vi "rqcAlice Delay Line Test (Low Level Example).vi"() -> ()   [LabVIEW 2018]
uses:
  FPGA/Alice/Custom Controls/Phase Modulator/rqcAlice Mod.Config.ctl
  Custom Controls/rqcAlice States.ctl
  FPGA/Alice/Custom Controls/Main State Machine/rqcAlice DAC Clock Positions.ctl
  Shared/Shared FPGA Lib/Shared Logic/Custom Controls/rqc Random Generator.parameters.ctl
  Shared/Shared FPGA Lib/Shared Logic/Custom Controls/rqc Random Generator.value type.ctl
  Shared/Shared Host Lib/rqc ServiceNET/Custom Controls/rqc ServiceNET command.ctl
  Shared/Shared Host Lib/rqc ServiceNET/Alice/Custom Controls/rqcAlice ServiceNET control.ctl
  <vilib>/FPGAPlugInAG/PCI-7811R/niLvFpga_Open_PCI-7811R.vi
  <vilib>/rvi/interface/common/dynamic/niFpgaDynamicAddResources.vi
  <vilib>/FPGAPlugInAG/Dynamic/niLvFpga_Close_Dynamic.vi
  <vilib>/rvi/interface/nirviOpenFPGA/nirviOpenFPGA.xnode
  FPGA Bitfiles/rqcAlice FPGA (7811R) v 2.3.0.lvbitx
  <vilib>/rvi/interface/nirviCloseFPGA/nirviCloseFPGA.xnode
panel:
  in  "Attenuation, dB":fxp<+,7,6>
  in  "SD/Coax Select":bool
  in  "RndGen.parameters":T1={"value type"=enum."constant", "constant"=150, "num of levels"=0, "levels values"=[0, 0, 0, 0]}
  in  "DAC Clock params":T3=[18, 38]
  out "XY Graph":T4(graph)={"appended array"=[49350.0, 49351.0, 49352.0, 49353.0, 49354.0, 49355.0, 49356.0, 49357.0, 49358.0, 49359.0, 49360.0, 49361.0, 49362.0, 49363.0, 49364.0, 49365.0, 49366.0, 49367.0, 49368.0, 49369.0, 49370.0, 49371.0, 49372.0, 49373.0, 49374.0, 49375.0, 49376.0, 49377.0, 49378.0, 49379.0, 49380.0, 49381.0, 49382.0, 49383.0, 49384.0, 49385.0, 49386.0, 49387.0, 49388.0, 49389.0, 49390.0, 49391.0, 49392.0, 49393.0, 49394.0, 49395.0, 49396.0, 49397.0, 49398.0, 49399.0, 49400.0, 49401.0, 49402.0, 49403.0, 49404.0, 49405.0, 49406.0, 49407.0, 49408.0, 49409.0, 49410.0, 49411.0, 49412.0, 49413.0, 49414.0, 49415.0, 49416.0, 49417.0, 49418.0, 49419.0, 49420.0, 49421.0, 49422.0, 49423.0, 49424.0, 49425.0, 49426.0, 49427.0, 49428.0, 49429.0, 49430.0, 49431.0, 49432.0, 49433.0, 49434.0, 49435.0], "appended array"=[4.0, 12.0, 24.0, 27.0, 45.0, 53.0, 39.0, 47.0, 36.0, 40.0, 40.0, 34.0, 37.0, 25.0, 9.0, 7.0, 2.0, 0.0, 0.0, 5.0, 8.0, 17.0, 20.0, 30.0, 49.0, 49.0, 43.0, 39.0, 48.0, 46.0, 47.0, 34.0, 29.0, 19.0, 9.0, 9.0, 1.0, 4.0, 3.0, 7.0, 5.0, 9.0, 23.0, 38.0, 37.0, 54.0, 30.0, 46.0, 51.0, 40.0, 47.0, 37.0, 33.0, 8.0, 5.0, 4.0, 3.0, 1.0, 3.0, 0.0, 3.0, 8.0, 15.0, 26.0, 33.0, 39.0, 45.0, 48.0, 54.0, 48.0, 44.0, 41.0, 43.0, 33.0, 20.0, 12.0, 9.0, 3.0, 2.0, 3.0, 5.0, 11.0, 19.0, 25.0, 34.0]}
  out "Delay Line Value":u32=49435
  in  "Delay Line Delta":u32=1
  in  "Delay Line max":u32=49450
  in  "Delay Line min":u32=49350
  out "error out":errorcluster
  in  "Stop":bool
  out "connected?":bool
  in  "port":u16=5020
  out "Current State":T5=enum."App.Stop"
  in  "Modulator config":T6={"mod.on"=9, "mod.off"=2}
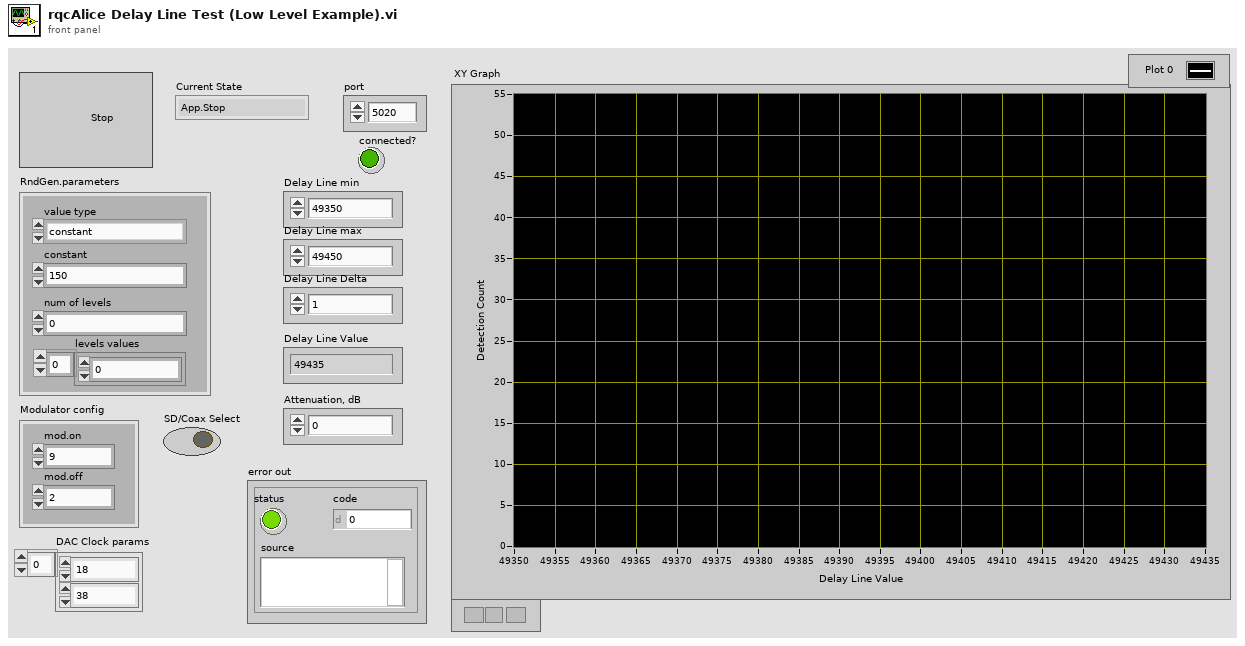
[diagram p1: front panel]
types:
  T1 = typedef "rqc Random Generator.parameters.ctl" = cluster{"value type":T2, "constant":u16, "num of levels":u16, "levels values":u16[]}
  T2 = typedef "rqc Random Generator.value type.ctl" = enum16{"random value", "constant"}
  T3 = typedef "rqcAlice DAC Clock Positions.ctl" = u8[]
  T4 = cluster{"appended array":dbl[], "appended array":dbl[]}
  T5 = typedef "rqcAlice States.ctl" = enum16{"HW.configure", "HW.meas", "NET.create", "NET.connect", "NET.readCommand", "NET.sendCommand", "NET.readData", "NET.close", "Meas.Start", "Meas.NextStep", "Meas.restart", "Meas.Done", "App.HandleEvent", "App.HandleError", "App.Stop"}
  T6 = typedef "rqcAlice Mod.Config.ctl" = cluster{"mod.on":u8, "mod.off":u8}
  T7 = typedef "rqc ServiceNET command.ctl" = enum8{"NONE", "READY", "START", "PING"}
  T8 = typedef "rqcAlice ServiceNET control.ctl" = cluster{"connection ID":refnum<k5>, "port":u16, "connected?":bool}
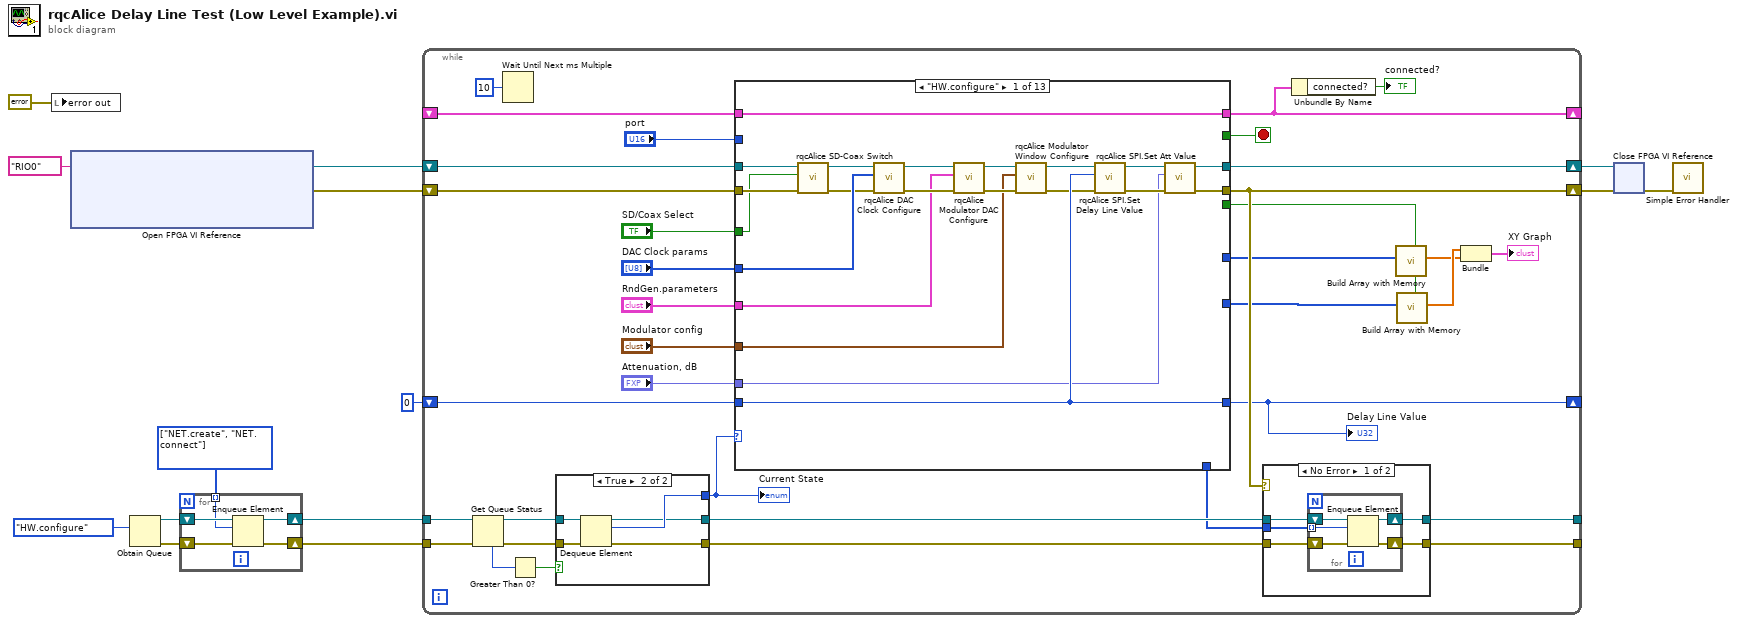
[diagram p0: block diagram]
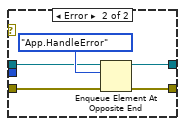
[diagram p2: hidden frame]
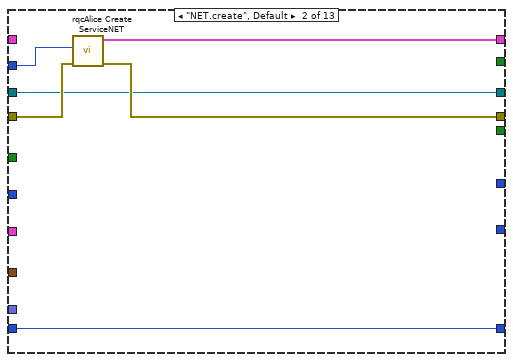
[diagram p3: hidden frame]
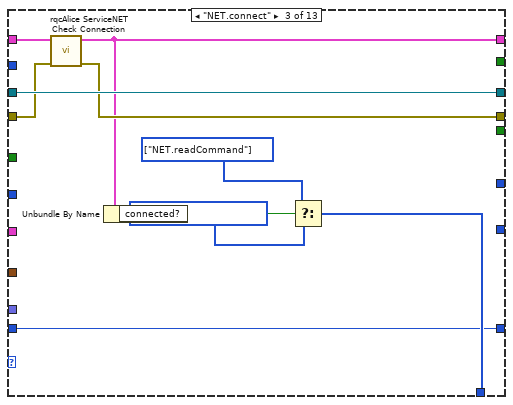
[diagram p4: hidden frame]
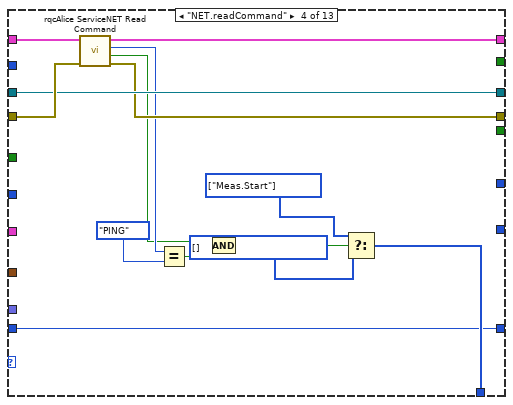
[diagram p5: hidden frame]
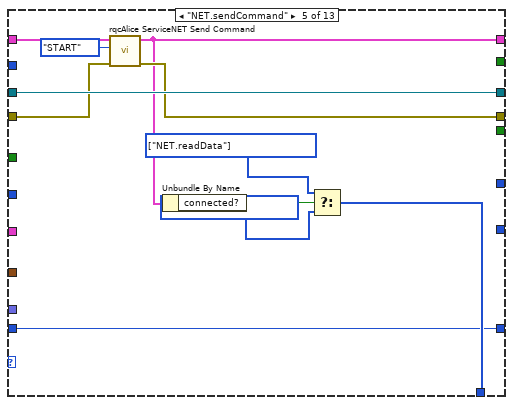
[diagram p6: hidden frame]
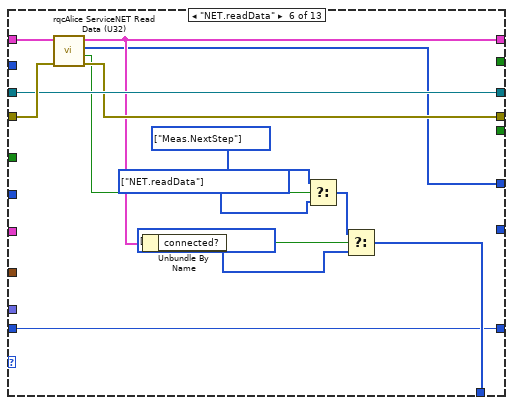
[diagram p7: hidden frame]
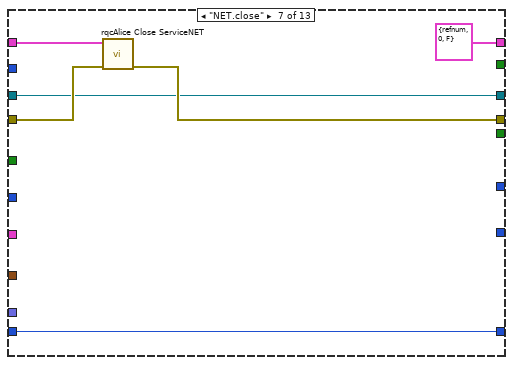
[diagram p8: hidden frame]
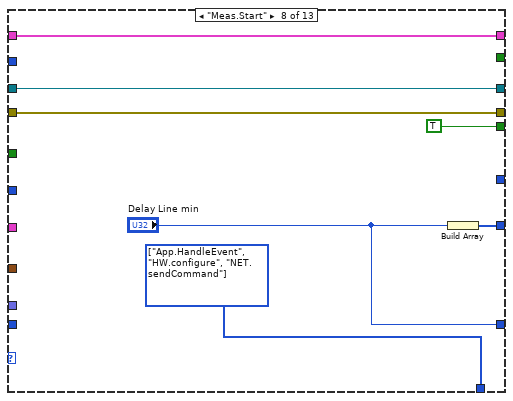
[diagram p9: hidden frame]
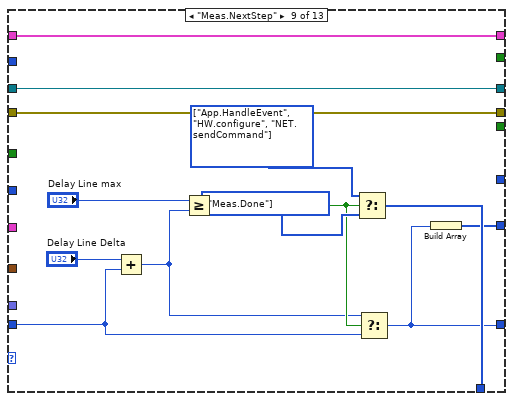
[diagram p10: hidden frame]
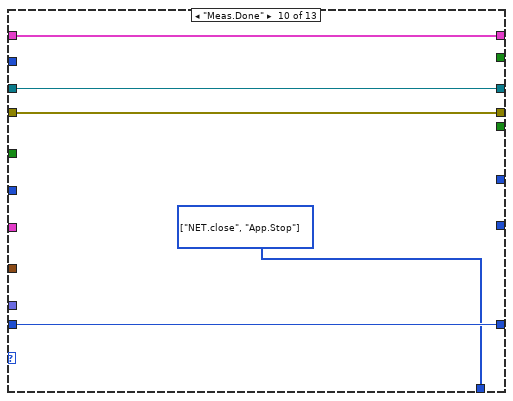
[diagram p11: hidden frame]
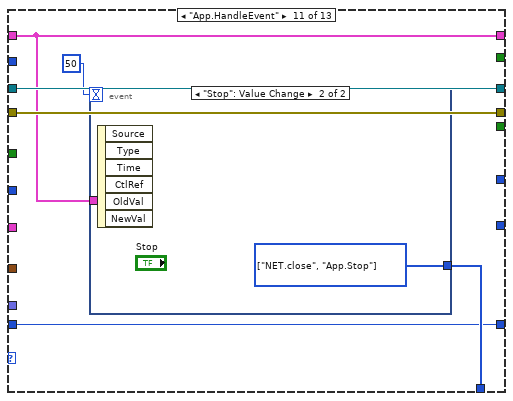
[diagram p12: hidden frame]
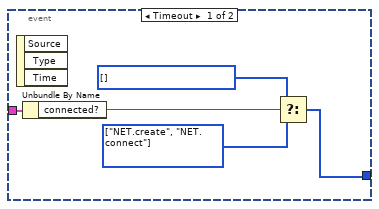
[diagram p13: hidden frame]
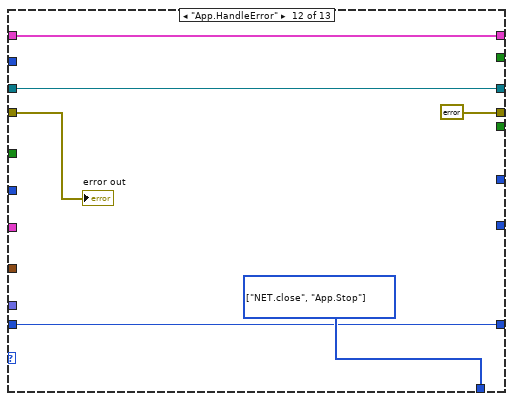
[diagram p14: hidden frame]
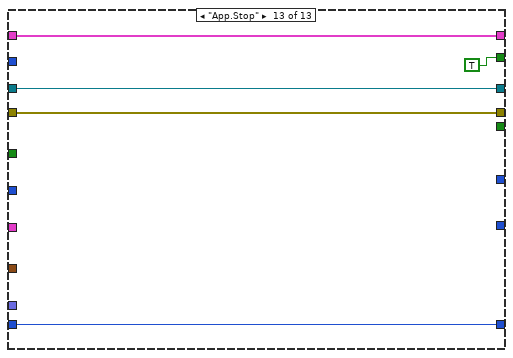
[diagram p15: hidden frame]
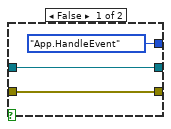
[diagram p16: hidden frame]
diagram:
  w6 = T5[] [enum."NET.create", enum."NET.connect"] items=["HW.configure", "HW.meas", "NET.create", "NET.connect", "NET.readCommand", "NET.sendCommand", "NET.readData", "NET.close", "Meas.Start", "Meas.NextStep", "Meas.restart", "Meas.Done", "App.HandleEvent", "App.HandleError", "App.Stop"]
  n1 = local write "error out"(errorcluster {"status"=FALSE, "code"=0, "source"=""} ("error out")) -> ()
  n2 = xnode "Open FPGA VI Reference"("resource name"=tag "RIO0") -> ("FPGA VI Reference Out"=w13:refnum<k20>, "error out"=w12:errorcluster)  [unwired: 1 in]
  n3 = Obtain Queue(element data type=rqcAlice_States."HW.configure" ("rqcAlice States")) -> (queue out=w8:refnum<queue>, error out=w7:errorcluster)  [unwired: 4 in, 1 out]
  n4 = for {
    shift-right: [w17] -> w5
    shift-left: w8 -> [w19]
    shift-right: [w16] -> w4
    shift-left: w7 -> [w18]
    tunnel: w6 -> [w15] mode=indexing
    n5 = Enqueue Element(queue=w19, element=w15, error in (no error)=w18) -> (queue out=w17:refnum<queue>, error out=w16:errorcluster)  [unwired: 1 in, 1 out]
  }
  n6 = while {
    tunnel: w5 -> [w50]
    shift-right: [w51] -> w11
    shift-left: w13 -> [w54]
    shift-right: [w43] -> w10
    shift-left: w12 -> [w53]
    tunnel: w4 -> [w49]
    tunnel: [w40] -> _
    tunnel: [w39] -> _
    shift-right: [w35] -> _
    shift-left: _ -> [w37]
    shift-right: [w29] -> _
    shift-left: u32 0 ("Delay Line min") -> [w31]
    stop <- w33 stop-if-true
    n7 = Get Queue Status(queue=w50, error in (no error)=w49) -> (queue out=w46:refnum<queue>, error out=w45:errorcluster, # elements in queue=w48:i32)  [unwired: 1 in, 5 out]
    n8 = Wait Until Next ms Multiple(millisecond multiple=u32 10) -> ()  [unwired: 1 out]
    n9 = Greater Than 0?(x=w48) -> (x > 0?=w47:bool)
    n10 = case shown="True" w47 {
      tunnel: w46 -> [w201 w207]
      tunnel: w45 -> [w200 w206]
      tunnel: [rqcAlice_States."App.HandleEvent" ("rqcAlice States") w205] -> w44
      tunnel: [w201 w204] -> w42
      tunnel: [w200 w203] -> w41
      frame False {
      }
      frame True {
        n11 = Dequeue Element(queue=w207, error in (no error)=w206) -> (queue out=w204:refnum<queue>, element=w205:T5, error out=w203:errorcluster)  [unwired: 1 in, 1 out]
      }
    }
    "Current State" <- w44
    n12 = case shown="\"HW.configure\"" w44 {
      tunnel: w54 -> [w82 w93 w106 w117 w131 w143 w147 w157 w170 w175 w182 w193 w198]
      tunnel: w53 -> [w81 w95 w104 w119 w129 w144 w150 w156 w169 w174 w181 w192 w197]
      tunnel: "Modulator config" -> [w86 _ _ _ _ _ _ _ _ _ _ _ _]
      tunnel: [w73 w93 w106 w117 w131 w143 w147 w157 w170 w175 w182 w193 w198] -> w51
      tunnel: [w71 w94 w103 w116 w128 w142 w149 w156 w169 w174 w181 errorcluster {"status"=FALSE, "code"=0, "source"=""} ("error out") w197] -> w43
      tunnel: [_ _ w99 w108 w122 w134 _ w155 w165 w172 w178 w190 _] -> w38
      tunnel: [w85 w96 w102 w118 w126 w141 T8 {"connection ID"=refnum, "port"=0, "connected?"=FALSE} ("rqcAlice ServiceNET out") w158 w171 w176 w179 w194 w196] -> w35
      tunnel: w37 -> [w85 _ w105 w120 w130 w145 w151 w158 w171 w176 w179 w194 w196]
      tunnel: "port" -> [_ w92 _ _ _ _ _ _ _ _ _ _ _]
      tunnel: [_ _ _ _ _ _ _ _ _ _ _ _ TRUE] -> w33
      tunnel: w31 -> [w76 w91 w97 w107 w121 w133 w146 _ w161 w173 w177 w189 w195]
      tunnel: [w76 w91 w97 w107 w121 w133 w146 "Delay Line min" w160 w173 w177 w189 w195] -> w29
      tunnel: [_ _ _ _ _ w132 _ _ _ _ _ _ _] -> w30
      tunnel: [_ _ _ _ _ _ _ w152 w159 _ _ _ _] -> w28
      tunnel: [_ _ _ _ _ _ _ TRUE _ _ _ _ _] -> w27
      tunnel: "DAC Clock params" -> [w84 _ _ _ _ _ _ _ _ _ _ _ _]
      tunnel: "RndGen.parameters" -> [w83 _ _ _ _ _ _ _ _ _ _ _ _]
      tunnel: "SD/Coax Select" -> [w78 _ _ _ _ _ _ _ _ _ _ _ _]
      tunnel: "Attenuation, dB" -> [w70 _ _ _ _ _ _ _ _ _ _ _ _]
      frame "HW.configure" {
        n13 = call "rqcAlice SD-Coax Switch.vi"("error in"=w81, "SD/Coax Select"=w78, "Alice FPGA Reference In"=w82) -> ("error out"=w79:errorcluster, "Alice FPGA Reference Out"=w80:refnum<k20>)  [unwired: 7 in]
        n14 = call "rqcAlice DAC Clock Configure.vi"("error in"=w79, "DAC Clock params"=w84, "Alice FPGA Reference In"=w80) -> ("error out"=w89:errorcluster, "Alice FPGA Reference Out"=w90:refnum<k20>)  [unwired: 7 in]
        n15 = call "rqcAlice Modulator DAC Configure.vi"("error in"=w89, "RndGen.parameters"=w83, "Alice FPGA Reference In"=w90) -> ("error out"=w87:errorcluster, "Alice FPGA Reference Out"=w88:refnum<k20>)  [unwired: 7 in]
        n16 = call "rqcAlice Modulator Window Configure.vi"("error in"=w87, "Modulator config"=w86, "Alice FPGA Reference In"=w88) -> ("error out"=w75:errorcluster, "Alice FPGA Reference Out"=w77:refnum<k20>)  [unwired: 7 in]
        n17 = call "rqcAlice SPI.Set Delay Line Value.vi"("error in"=w75, "Delay Line Value"=w76, "Alice FPGA Reference In"=w77) -> ("error out"=w72:errorcluster, "Alice FPGA Reference Out"=w74:refnum<k20>)  [unwired: 7 in]
        n18 = call "rqcAlice SPI.Set Att Value.vi"("error in"=w72, "Attenuation, dB"=w70, "Alice FPGA Reference In"=w74) -> ("error out"=w71:errorcluster, "Alice FPGA Reference Out"=w73:refnum<k20>)  [unwired: 7 in]
      }
      frame "NET.create", Default {
        n19 = call "rqcAlice Create ServiceNET.vi"("error in"=w95, "port"=w92) -> ("error out"=w94:errorcluster, "rqcAlice ServiceNET control"=w96:T8)  [unwired: 8 in]
      }
      frame "NET.connect" {
        w98 = T5[] [] items=["HW.configure", "HW.meas", "NET.create", "NET.connect", "NET.readCommand", "NET.sendCommand", "NET.readData", "NET.close", "Meas.Start", "Meas.NextStep", "Meas.restart", "Meas.Done", "App.HandleEvent", "App.HandleError", "App.Stop"] ("f")
        w100 = T5[] [enum."NET.readCommand"] items=["HW.configure", "HW.meas", "NET.create", "NET.connect", "NET.readCommand", "NET.sendCommand", "NET.readData", "NET.close", "Meas.Start", "Meas.NextStep", "Meas.restart", "Meas.Done", "App.HandleEvent", "App.HandleError", "App.Stop"]
        n20 = call "rqcAlice ServiceNET Check Connection.vi"("error in"=w104, "rqcAlice ServiceNET in"=w105) -> ("error out"=w103:errorcluster, "rqcAlice ServiceNET out"=w102:T8)  [unwired: 8 in]
        n21 = Unbundle By Name(w102) -> ("connected?"=w101:bool)
        n22 = Select(t=w100, s=w101, f=w98) -> (s? t:f=w99:T5[])
      }
      frame "NET.readCommand" {
        w109 = T5[] [] items=["HW.configure", "HW.meas", "NET.create", "NET.connect", "NET.readCommand", "NET.sendCommand", "NET.readData", "NET.close", "Meas.Start", "Meas.NextStep", "Meas.restart", "Meas.Done", "App.HandleEvent", "App.HandleError", "App.Stop"] ("f")
        w110 = T5[] [enum."Meas.Start"] items=["HW.configure", "HW.meas", "NET.create", "NET.connect", "NET.readCommand", "NET.sendCommand", "NET.readData", "NET.close", "Meas.Start", "Meas.NextStep", "Meas.restart", "Meas.Done", "App.HandleEvent", "App.HandleError", "App.Stop"] ("f")
        n23 = call "rqcAlice ServiceNET Read Command.vi"("error in"=w119, "rqcAlice ServiceNET in"=w120) -> ("error out"=w116:errorcluster, "cmd valid"=w112:bool, "command"=w114:T7, "rqcAlice ServiceNET out"=w118:T8)  [unwired: 6 in]
        n24 = Equal?(x=w114, y=rqc_ServiceNET_command."PING" ("command")) -> (x = y?=w113:bool)
        n25 = Compound Arithmetic op=AND(w112, w113) -> (w111:bool)
        n26 = Select(t=w110, s=w111, f=w109) -> (s? t:f=w108:T5[])
      }
      frame "NET.sendCommand" {
        w123 = T5[] [] items=["HW.configure", "HW.meas", "NET.create", "NET.connect", "NET.readCommand", "NET.sendCommand", "NET.readData", "NET.close", "Meas.Start", "Meas.NextStep", "Meas.restart", "Meas.Done", "App.HandleEvent", "App.HandleError", "App.Stop"] ("f")
        w124 = T5[] [enum."NET.readData"] items=["HW.configure", "HW.meas", "NET.create", "NET.connect", "NET.readCommand", "NET.sendCommand", "NET.readData", "NET.close", "Meas.Start", "Meas.NextStep", "Meas.restart", "Meas.Done", "App.HandleEvent", "App.HandleError", "App.Stop"] ("f")
        n27 = call "rqcAlice ServiceNET Send Command.vi"("error in"=w129, "command"=rqc_ServiceNET_command."START", "rqcAlice ServiceNET in"=w130) -> ("error out"=w128:errorcluster, "rqcAlice ServiceNET out"=w126:T8)  [unwired: 7 in]
        n28 = Unbundle By Name(w126) -> ("connected?"=w125:bool)
        n29 = Select(t=w124, s=w125, f=w123) -> (s? t:f=w122:T5[])
      }
      frame "NET.readData" {
        w135 = T5[] [] items=["HW.configure", "HW.meas", "NET.create", "NET.connect", "NET.readCommand", "NET.sendCommand", "NET.readData", "NET.close", "Meas.Start", "Meas.NextStep", "Meas.restart", "Meas.Done", "App.HandleEvent", "App.HandleError", "App.Stop"] ("f")
        w140 = T5[] [enum."Meas.NextStep"] items=["HW.configure", "HW.meas", "NET.create", "NET.connect", "NET.readCommand", "NET.sendCommand", "NET.readData", "NET.close", "Meas.Start", "Meas.NextStep", "Meas.restart", "Meas.Done", "App.HandleEvent", "App.HandleError", "App.Stop"] ("t")
        w138 = T5[] [enum."NET.readData"] items=["HW.configure", "HW.meas", "NET.create", "NET.connect", "NET.readCommand", "NET.sendCommand", "NET.readData", "NET.close", "Meas.Start", "Meas.NextStep", "Meas.restart", "Meas.Done", "App.HandleEvent", "App.HandleError", "App.Stop"] ("f")
        n30 = call "rqcAlice ServiceNET Read Data (U32).vi"("error in"=w144, "rqcAlice ServiceNET in"=w145) -> ("error out"=w142:errorcluster, "data valid"=w139:bool, "data"=w132:u32[], "rqcAlice ServiceNET out"=w141:T8)  [unwired: 6 in]
        n31 = Unbundle By Name(w141) -> ("connected?"=w137:bool)
        n32 = Select(t=w140, s=w139, f=w138) -> (s? t:f=w136:T5[])
        n33 = Select(t=w136, s=w137, f=w135) -> (s? t:f=w134:T5[])
      }
      frame "NET.close" {
        n34 = call "rqcAlice Close ServiceNET.vi"("error in"=w150, "rqcAlice ServiceNET in"=w151) -> ("error out"=w149:errorcluster)  [unwired: 9 in]
      }
      frame "Meas.Start" {
        w155 = T5[] [enum."App.HandleEvent", enum."HW.configure", enum."NET.sendCommand"] items=["HW.configure", "HW.meas", "NET.create", "NET.connect", "NET.readCommand", "NET.sendCommand", "NET.readData", "NET.close", "Meas.Start", "Meas.NextStep", "Meas.restart", "Meas.Done", "App.HandleEvent", "App.HandleError", "App.Stop"] ("f")
        n35 = Build Array("Delay Line min") -> (w152:u32[])
      }
      frame "Meas.NextStep" {
        w164 = T5[] [enum."Meas.Done"] items=["HW.configure", "HW.meas", "NET.create", "NET.connect", "NET.readCommand", "NET.sendCommand", "NET.readData", "NET.close", "Meas.Start", "Meas.NextStep", "Meas.restart", "Meas.Done", "App.HandleEvent", "App.HandleError", "App.Stop"] ("f")
        w166 = T5[] [enum."App.HandleEvent", enum."HW.configure", enum."NET.sendCommand"] items=["HW.configure", "HW.meas", "NET.create", "NET.connect", "NET.readCommand", "NET.sendCommand", "NET.readData", "NET.close", "Meas.Start", "Meas.NextStep", "Meas.restart", "Meas.Done", "App.HandleEvent", "App.HandleError", "App.Stop"] ("f")
        n36 = Add(x="Delay Line Delta", y=w161) -> (x+y=w162:u32)
        n37 = Greater Or Equal?(x="Delay Line max", y=w162) -> (x >= y?=w163:bool)
        n38 = Select(t=w166, s=w163, f=w164) -> (s? t:f=w165:T5[])
        n39 = Select(t=w162, s=w163, f=w161) -> (s? t:f=w160:u32)
        n40 = Build Array(w160) -> (w159:u32[])
      }
      frame "Meas.Done" {
        w172 = T5[] [enum."NET.close", enum."App.Stop"] items=["HW.configure", "HW.meas", "NET.create", "NET.connect", "NET.readCommand", "NET.sendCommand", "NET.readData", "NET.close", "Meas.Start", "Meas.NextStep", "Meas.restart", "Meas.Done", "App.HandleEvent", "App.HandleError", "App.Stop"] ("f")
      }
      frame "App.HandleEvent" {
        n41 = event shown="[1] \"Stop\": Value Change" {
          selector: _ -> [_ _]
          dyn-events: _ -> [_ _]
          timeout: 50 -> [_ _]
          tunnel: w179 -> [w187 _]
          tunnel: [w183 w188] -> w178
          event Timeout {
            w184 = T5[] [enum."NET.create", enum."NET.connect"] items=["HW.configure", "HW.meas", "NET.create", "NET.connect", "NET.readCommand", "NET.sendCommand", "NET.readData", "NET.close", "Meas.Start", "Meas.NextStep", "Meas.restart", "Meas.Done", "App.HandleEvent", "App.HandleError", "App.Stop"]
            w185 = T5[] [] items=["HW.configure", "HW.meas", "NET.create", "NET.connect", "NET.readCommand", "NET.sendCommand", "NET.readData", "NET.close", "Meas.Start", "Meas.NextStep", "Meas.restart", "Meas.Done", "App.HandleEvent", "App.HandleError", "App.Stop"]
            n42 = event-data() -> ()  [unwired: 1 in, 3 out]
            n43 = Unbundle By Name(w187) -> ("connected?"=w186:bool)
            n44 = Select(t=w185, s=w186, f=w184) -> (s? t:f=w183:T5[])
          }
          event "Stop": Value Change {
            w188 = T5[] [enum."NET.close", enum."App.Stop"] items=["HW.configure", "HW.meas", "NET.create", "NET.connect", "NET.readCommand", "NET.sendCommand", "NET.readData", "NET.close", "Meas.Start", "Meas.NextStep", "Meas.restart", "Meas.Done", "App.HandleEvent", "App.HandleError", "App.Stop"]
            n45 = event-data() -> ()  [unwired: 1 in, 6 out]
          }
        }
      }
      frame "App.HandleError" {
        w190 = T5[] [enum."NET.close", enum."App.Stop"] items=["HW.configure", "HW.meas", "NET.create", "NET.connect", "NET.readCommand", "NET.sendCommand", "NET.readData", "NET.close", "Meas.Start", "Meas.NextStep", "Meas.restart", "Meas.Done", "App.HandleEvent", "App.HandleError", "App.Stop"] ("f")
        "error out" <- w192
      }
      frame "App.Stop" {
      }
    }
    "Delay Line Value" <- w29
    n46 = case shown="No Error" w43 {
      tunnel: w42 -> [w59 w68]
      tunnel: w41 -> [w58 w66]
      tunnel: [w57 w67] -> w40
      tunnel: [w56 w65] -> w39
      tunnel: w38 -> [w55 _]
      frame No Error {
        n47 = for {
          shift-right: [w62] -> w57
          shift-left: w59 -> [w64]
          shift-right: [w61] -> w56
          shift-left: w58 -> [w63]
          tunnel: w55 -> [w60] mode=indexing
          n48 = Enqueue Element(queue=w64, element=w60, error in (no error)=w63) -> (queue out=w62:refnum<queue>, error out=w61:errorcluster)  [unwired: 1 in, 1 out]
        }
      }
      frame Error {
        n49 = Enqueue Element At Opposite End(queue=w68, element=rqcAlice_States."App.HandleError" ("rqcAlice States"), error in (no error)=w66) -> (queue out=w67:refnum<queue>, error out=w65:errorcluster)  [unwired: 1 in, 1 out]
      }
    }
    n50 = Unbundle By Name(w35) -> ("connected?"=→"connected?":bool)
    n51 = call "Build Array with Memory.vi"("reset"=w27, "new array"=w30) -> ("appended array"=w24:dbl[])  [unwired: 9 in]
    n52 = call "Build Array with Memory.vi"("reset"=w27, "new array"=w28) -> ("appended array"=w25:dbl[])  [unwired: 9 in]
    n53 = Bundle("appended array"=w25, "appended array"=w24) -> (→"XY Graph":T4)  [unwired: 1 in]
  }
  n54 = xnode "Close FPGA VI Reference"("FPGA VI Reference In"=w11, "error in"=w10) -> ("error out"=w3:errorcluster)
  n55 = call <vilib>:"Simple Error Handler.vi"("error in (no error)"=w3) -> ()  [unwired: 4 in, 5 out]
